vi "TEST _Spec_LUT.vi"() -> ()   [LabVIEW 2024]
doc: "This VI is used to test the Spec LUT (Look Up Table) Select ChA!ChB and Drain!Fill\nShould produce the spec index for the level entered.\nNote: Meausre shows the value whre Measure R is enabled."
uses:
  Control Definitions/Def Spec RNG.ctl
  Control Definitions/Ded LUT_Status.ctl
  Control Definitions/Def FullCfg.ctl
  Control Definitions/Def BenchCfg.ctl
  Control Definitions/Def PumpCtlRefs.ctl
  Control Definitions/Def_PumpSpeed.ctl
  Control Definitions/Def Bench Status.ctl
panel:
  in  "Full Cfg 2":T1={"Bench Config"={"Name"="OLR001", {"Step Levels"=0.05, "Tolerance"=0.01, "Sample Rate"=0.05, "Resistor"=100.0, "M Level Cal"=1.0, "[B Level Cal"=0.0, "Max Fill Rate"=0.002, "Empty Inches"=8.0, "Full Inches"=2.6}}, "Test Value Table "=[[98.0, 102.0, 8.5, 8.5, 8.5, 8.5, 98.0, 102.0, 8.5, 8.5, 8.5, 8.5], [98.0, 102.0, 7.91, 8.01, 7.55, 7.65, 98.0, 102.0, 7.685, 7.785, 7.325, 7.425], [197.0, 203.0, 7.46, 7.56, 7.1, 7.2, 197.0, 203.0, 7.235, 7.335, 6.875, 6.975], [296.0, 304.0, 7.01, 7.11, 6.65, 6.75, 296.0, 304.0, 6.785, 6.885, 6.425, 6.525], [395.0, 405.0, 6.56, 6.66, 6.2, 6.3, 395.0, 405.0, 6.335, 6.435, 5.975, 6.075], [494.0, 506.0, 6.11, 6.21, 5.75, 5.85, 494.0, 506.0, 5.885, 5.985, 5.525, 5.625], [593.0, 607.0, 5.66, 5.76, 5.3, 5.4, 593.0, 607.0, 5.435, 5.535, 5.075, 5.175], [692.0, 708.0, 5.21, 5.31, 4.85, 4.95, 692.0, 708.0, 4.985, 5.085, 4.625, 4.725], [791.0, 809.0, 4.76, 4.86, 4.4, 4.5, 791.0, 809.0, 4.535, 4.635, 4.175, 4.275], [890.0, 910.0, 4.31, 4.41, 3.95, 4.05, 890.0, 910.0, 4.085, 4.185, 3.725, 3.825], [989.0, 1011.0, 3.86, 3.96, 3.5, 3.6, 989.0, 1011.0, 3.635, 3.735, 3.275, 3.375], [1088.0, 1112.0, 3.41, 3.51, 3.05, 3.15, 1088.0, 1112.0, 3.185, 3.285, 2.825, 2.925], [1088.0, 1112.0, 2.5, 2.5, 2.5, 2.5, 1088.0, 1112.0, 2.5, 2.5, 2.5, 2.5]], "Table Col Titles"=[["Aohm Lo", "Aohm Hi", "A Fill Lo", "A Fill Hi", "A Drain Lo", "A Drain Hi", "Bohm Lo", "Bohm Hi", "B Fill Lo", "B Fill Hi", "B Drain Lo", "B Drain Hi"]], "cluster"={"Fill "=refnum, "Drain"=refnum, "Level PV"=refnum, "Pump Speed"=refnum, "Run Test"=refnum, "Sim"=refnum, "Jog"=refnum, "Level SP"=refnum}, "Bench Status"={"Pump Status"=refnum, "Instrumnet\n Status"=refnum}}
  in  "stop":bool
  in  "Index":i32=3
  out "Set Point":dbl
  out "Spec Range Out":T5
  out "Measure":dbl
  in  "Drain!Fill":bool
  in  "Level IN inches":dbl
  in  "ChA/!ChB":bool
  # "Spec Lo(n)\n\nSpec Lo(n)\n\nSpec  Lo(n-1)"
  # "FILL LOGIC\nIn Range =    Spec Lo (n-1)  > Level > Spec Lo (n) \nSwitch Range =  Spec Hi (n) > Level > Spec Lo (n)\nMeausre R =  Level = {Spec Hi (n)  + Spec Lo (n-1)}/2 +/- 0.01 \nValid R = Spec Lo (n-1) > Level > Spec Hi (n)\nSet Point = Spec Lo(n)\n\nDRAIN LOGIC\nIn Range =  Spec Lo (n+1) > Level > Spec Lo (n)\nSwitch Range =  Spec Hi (n) > Level > Spec Lo (n)\nMeausre R =  Level = {Spec Hi (n)  + Spec Lo (n+1)}/2 +/- 0.01 \nValid R = Spec Lo (n+1) > Level > Spec Hi (n)\nSet Point = Spec Hi(n)"
  # "Use TEST_Spec_LUT.vi to test this logic\nTest Cases are tabulated in Level Rig ATP OLS-001 Config1.xlsx \n\ni   Ohm SwP   ATP   Measure\n2A  200\t  7.51\t7.46\t  7.735\t7.812"
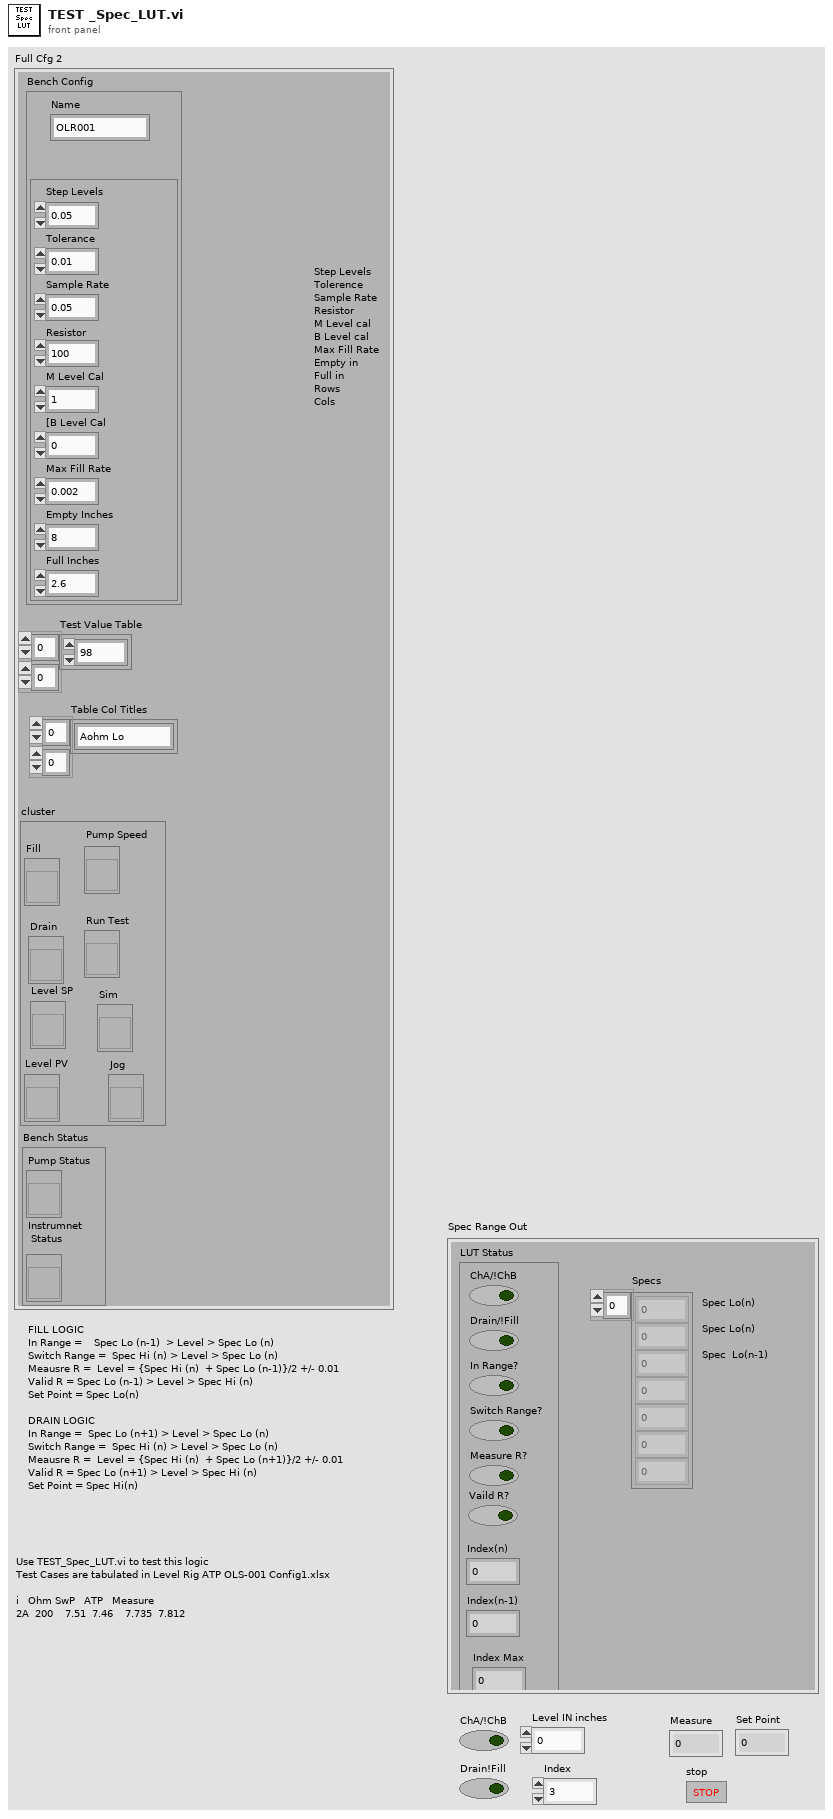
[diagram p1: front panel]
types:
  T1 = typedef "Def FullCfg.ctl" = cluster{"Bench Config":T2, "Test Value Table ":dbl[][], "Table Col Titles":string[][], "cluster":T3, "Bench Status":T4}
  T2 = typedef "Def BenchCfg.ctl" = cluster{"Name":string, cluster{"Step Levels":dbl, "Tolerance":dbl, "Sample Rate":dbl, "Resistor":dbl, "M Level Cal":dbl, "[B Level Cal":dbl, "Max Fill Rate":dbl, "Empty Inches":dbl, "Full Inches":dbl}}
  T3 = typedef "Def PumpCtlRefs.ctl" = cluster{"Fill ":refnum<vi>, "Drain":refnum<vi>, "Level PV":refnum<vi>, "Pump Speed":refnum<vi>, "Run Test":refnum<vi>, "Sim":refnum<vi>, "Jog":refnum<vi>, "Level SP":refnum<vi>}
  T4 = typedef "Def Bench Status.ctl" = cluster{"Pump Status":refnum<vi>, "Instrumnet\n Status":refnum<vi>}
  T5 = typedef "Def Spec RNG.ctl" = cluster{"Specs":dbl[], "LUT Status":T6}
  T6 = typedef "Ded LUT_Status.ctl" = cluster{"ChA/!ChB":bool, "Drain/!Fill":bool, "In Range?":bool, "Switch Range?":bool, "Measure R?":bool, "Vaild R?":bool, "Index(n)":i32, "Index(n-1)":i32, "Index Max":i32}
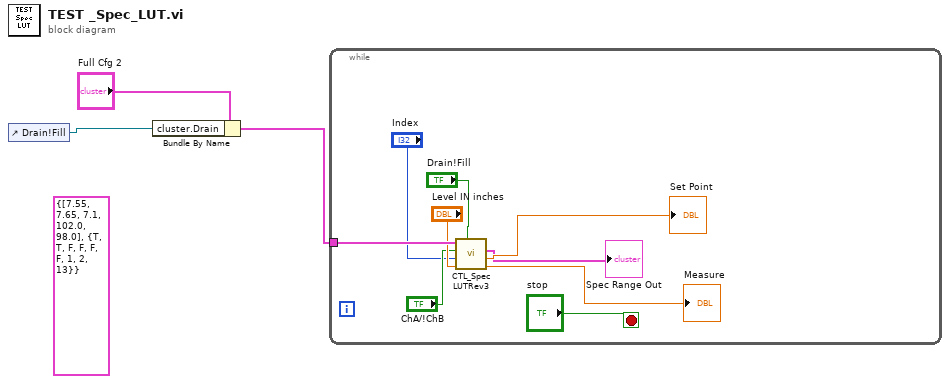
[diagram p0: block diagram]
diagram:
  (unwired) T5 {"Specs"=[7.55, 7.65, 7.1, 102.0, 98.0], "LUT Status"={"ChA/!ChB"=TRUE, "Drain/!Fill"=TRUE, "In Range?"=FALSE, "Switch Range?"=FALSE, "Measure R?"=FALSE, "Vaild R?"=FALSE, "Index(n)"=1, "Index(n-1)"=2, "Index Max"=13}} ("Spec Range Out")
  n1 = control-ref of="Drain!Fill"() -> (w2:refnum<vi>)
  n2 = Bundle By Name(cluster="Full Cfg 2", "cluster.Drain"=w2) -> (w3:T1)
  n3 = while {
    tunnel: w3 -> [w12]
    stop <- "stop" stop-if-true
    n4 = call "CTL_Spec LUTRev3.vi"("Drain!Fill"="Drain!Fill", "Level IN inches"="Level IN inches", "Index"="Index", "ChA/!ChB"="ChA/!ChB", "Full Cfg"=w12) -> ("Level Out"=→"Measure":dbl, "Set Point"=→"Set Point":dbl, "Spec Range Out"=→"Spec Range Out":T5)  [unwired: 3 in, 1 out]
  }
